vi "Read Analogue.vi"(8 "error in (no error)":errorcluster, 11 "Abstract DMM in":refnum<class "DMM Instrument.lvclass">) -> (0 "error out":errorcluster, 2 "Waveforms":waveform(dbl)[](array[waveform]), 3 "Abstract DMM out":refnum<class "DMM Instrument.lvclass">)   [LabVIEW 2025, in "DMM.lvlib" / "DMM Instrument.lvclass"]
uses:
  DMM Instrument.lvclass
  DMM Instrument.lvclass/DMM Instrument.ctl
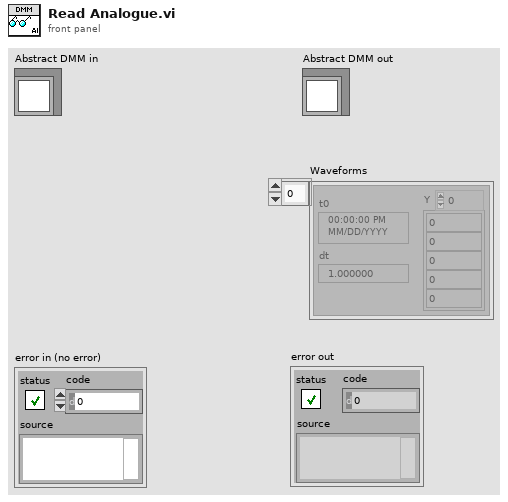
[diagram p1: front panel]
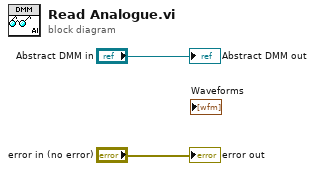
[diagram p0: block diagram]
diagram:
  "error out" <- "error in (no error)"
  "Abstract DMM out" <- "Abstract DMM in"
